vi "Get roboRIO PIDs.vi"() -> (3 "roboRIO PIDs":u32[](array[numeric]) format="%.0x")   [LabVIEW 2021]
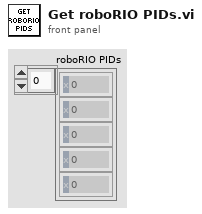
[diagram p1: front panel]
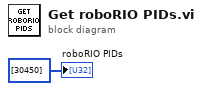
[diagram p0: block diagram]
diagram:
  "roboRIO PIDs" <- u32[] [30450]
